vi "String Array to String with Commas.vi"(10 "Array":string[](array[string])) -> (2 "String":string)   [LabVIEW 2020, in "Data.PG.lvclass"]
uses:
  Data.PG.lvclass
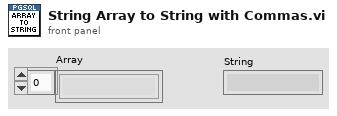
[diagram p1: front panel]
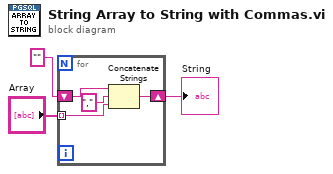
[diagram p0: block diagram]
diagram:
  n1 = for {
    tunnel: "Array" -> [w4] mode=indexing
    shift-right: [w7] -> w1
    shift-left: "" -> [w6]
    n2 = Concatenate Strings(w6, "," ("string"), w4) -> (w7:string)
  }
  "String" <- w1
